vi "FPGA_PPG_query_command.vi"(0 "resource_in":refnum<visa-resource-name>, 2 "mem_addr":u32, 5 "error in (no error)":errorcluster) -> (14 "resource_out":refnum<visa-resource-name>, 16 "command":string, 19 "error out":errorcluster)   [LabVIEW 2014, in "NI-FPGA_PPG_Driver.lvlib"]
doc: "Queries the command specified by the address.\n\nContact: Falk Ziegler, eMail: ziegler@physik.uni-greifswald.de"
uses:
  NI-FPGA_PPG_Driver.lvlib
  <vilib>/rvi/interface/nirviReadWriteControl/nirviReadWriteControl.xnode
  <vilib>/rvi/interface/nirviMethod/nirviMethod.xnode
  FPGA_PPG_action_type.ctl
  FPGA_PPG_error_type.ctl
  FPGA_PPG_vi_ref.ctl
  D:/Workspace/PyCharm/Tilda/TildaTarget/Labview14/FPGA Bitfiles/TiTaProj_COF_PPG_100MHz.lvbitx
  <vilib>/rvi/errors/niLvFpgaMergeErrorWithErrorCode.vi
panel:
  in  "errorCodes":T1=enum."can't change state while pattern output is in progress"
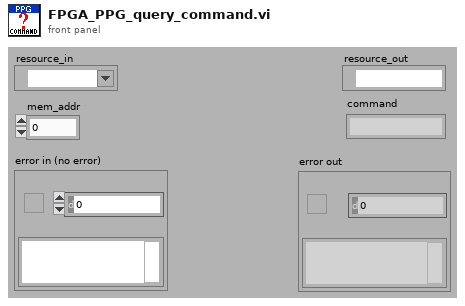
[diagram p1: front panel]
types:
  T1 = typedef "NI-FPGA_PPG_Driver.lvlib/FPGA_PPG_error_type.ctl" = enum16{"no error", "resource not initialized (no commands and invalid mem address)", "wrong memory address (address > Nof commands)", "invalid time value (probably too short)", "cannot start FPGA because one or more errors occured", "FIFO (internal) empty unexpectedly", "DMA FIFO (download from host) full unexpectedly", "checking number of commands: failed", "unknown error 8", "unknown error 9", "unknown error 10", "unknown error 11", "unknown error 12", "unknown error 13", "unknown error 14", "unknown error 15", "unknown error 16", "unknown error 17", "unknown error 18", "unknown error 19", "can't change state while pattern output is in progress"}
  T2 = typedef "NI-FPGA_PPG_Driver.lvlib/FPGA_PPG_action_type.ctl" = enum16{"GET", "SET", "REMOVE"}
  T3 = typedef "NI-FPGA_PPG_Driver.lvlib/FPGA_PPG_vi_ref.ctl" = refnum<k20>
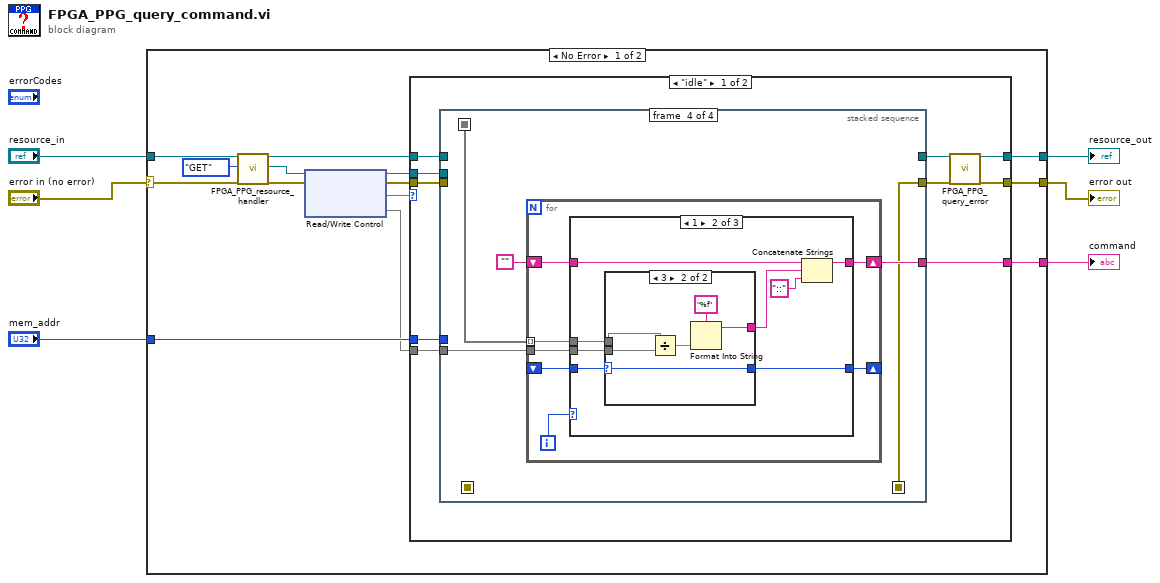
[diagram p0: block diagram]
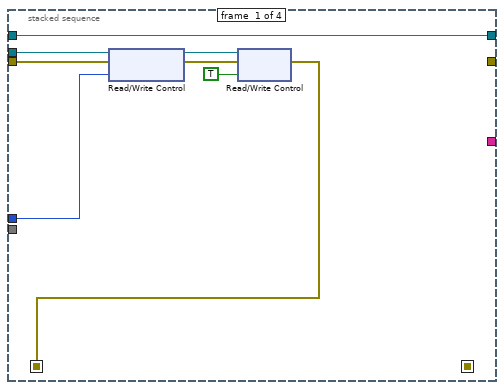
[diagram p2: hidden frame]
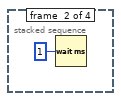
[diagram p3: hidden frame]
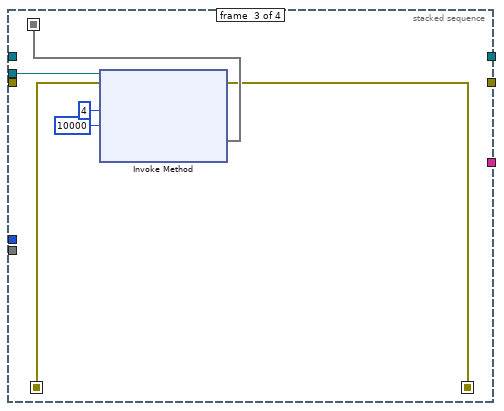
[diagram p4: hidden frame]
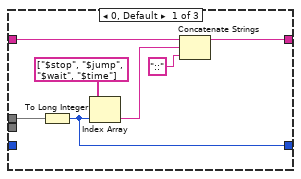
[diagram p5: hidden frame]
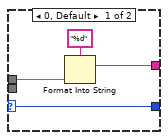
[diagram p6: hidden frame]
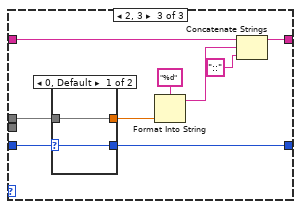
[diagram p7: hidden frame]
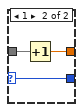
[diagram p8: hidden frame]
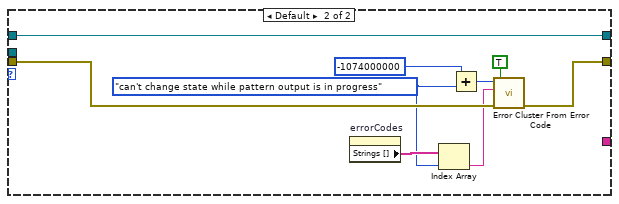
[diagram p9: hidden frame]
diagram:
  n1 = case shown="No Error" "error in (no error)" {
    selector: "error in (no error)" -> [w19 w107]
    tunnel: [w10 w107] -> w5
    tunnel: "resource_in" -> [w20 w106]
    tunnel: [w11 w106] -> w3
    tunnel: "mem_addr" -> [w13 _]
    tunnel: [w12 _] -> w1
    frame No Error {
      n2 = call "FPGA_PPG_resource_handler.vi"("resource_in"=w20, "action"=FPGA_PPG_action_type."GET", "error in (no error)"=w19) -> ("resource_out"=w16:refnum<visa-resource-name>, "FPGA VI Reference Out"=w8:T3, "error out"=w18:errorcluster)  [unwired: 14 in]
      n3 = xnode ("Read/Write Control")("FPGA VI Reference In"=w8, "error in"=w18) -> ("FPGA VI Reference Out"=w15:T3, "error out"=w14:errorcluster, "state"=w17, "ticks_per_us"=w7)
      n4 = case shown="\"idle\"" w17 {
        tunnel: w16 -> [w27 w105]
        tunnel: w15 -> [w30 _]
        tunnel: w14 -> [w29 w104]
        tunnel: [w24 w105] -> w11
        tunnel: w13 -> [w28 _]
        tunnel: [w26 _] -> w12
        tunnel: [w23 w102] -> w10
        tunnel: w7 -> [w21 _]
        frame "idle" {
          n5 = stacked-sequence {
            seq-local: [w31 _ _ _] -> [_ _ w44 _]
            seq-local: [_ _ w41 _] -> [_ _ _ w50]
            seq-local: [_ _ w40 _] -> [_ _ _ w47]
            tunnel: w30 -> [w38 _ w45 _]
            tunnel: w29 -> [w37 _ _ _]
            tunnel: w28 -> [w36 _ _ _]
            tunnel: w27 -> [w32 _ _ _]
            tunnel: [w32 _ _ _] -> w25
            tunnel: [_ _ _ w48] -> w26
            tunnel: [_ _ _ w47] -> w22
            tunnel: w21 -> [_ _ _ w46]
            frame #0 {
              n6 = xnode ("Read/Write Control")("FPGA VI Reference In"=w38, "error in"=w37, "mem_addr"=w36) -> ("FPGA VI Reference Out"=w35:T3, "error out"=w34:errorcluster)
              n7 = xnode ("Read/Write Control")("FPGA VI Reference In"=w35, "error in"=w34, "query"=TRUE) -> ("error out"=w31:errorcluster)  [unwired: 1 out]
            }
            frame #1 {
              n8 = Wait (ms)(milliseconds to wait=u32 1) -> ()  [unwired: 1 out]
            }
            frame #2 {
              n9 = xnode ("Invoke Method")("FPGA VI Reference In"=w45, "error in"=w44, "Number of Elements"=u32 4, "Timeout (ms)"=10000) -> ("error out"=w40:errorcluster, "Data"=w41:void[])  [unwired: 2 out]
            }
            frame #3 {
              n10 = for {
                tunnel: w50 -> [w56] mode=indexing
                shift-right: [w54] -> w48
                shift-left: "" ("Empty String Constant") -> [w55]
                shift-right: [w52] -> _
                shift-left: _ -> [w53]
                tunnel: w46 -> [w51]
                i -> [w57]
                n11 = case shown="1" w57 {
                  tunnel: w56 -> [w61 w68 w85]
                  tunnel: w55 -> [w63 w72 w89]
                  tunnel: [w62 w70 w87] -> w54
                  tunnel: [w58 w66 w83] -> w52
                  tunnel: w53 -> [_ w69 w86]
                  tunnel: w51 -> [_ w65 _]
                  frame 0, Default {
                    n12 = To Long Integer(number=w61) -> (32bit integer=w58:i32)
                    n13 = Index Array(array=string[] ["$stop", "$jump", "$wait", "$time"], index=w58) -> (element=w60:string)
                    n14 = Concatenate Strings(w63, w60, "::" ("string")) -> (w62:string)
                  }
                  frame 1 {
                    n15 = case shown="3" w69 {
                      selector: w69 -> [w73 w78]
                      tunnel: w68 -> [w75 w82]
                      tunnel: [w74 w79] -> w67
                      tunnel: [w73 w78] -> w66
                      tunnel: w65 -> [_ w77]
                      frame 0, Default {
                        n16 = Format Into String(format string="%d", w75) -> (resulting string=w74:string)  [unwired: 2 in, 1 out]
                      }
                      frame 3 {
                        n17 = Divide(x=w82, y=w77) -> (x/y=w80:dbl)
                        n18 = Format Into String(format string="%f", w80) -> (resulting string=w79:string)  [unwired: 2 in, 1 out]
                      }
                    }
                    n19 = Concatenate Strings(w72, w67, "::" ("string")) -> (w70:string)
                  }
                  frame 2, 3 {
                    n20 = case shown="0, Default" w86 {
                      selector: w86 -> [w92 w94]
                      tunnel: w85 -> [w93 w95]
                      tunnel: [w93 w96] -> w84
                      tunnel: [w92 w94] -> w83
                      frame 0, Default {
                      }
                      frame 1 {
                        n21 = Increment(x=w95) -> (x+1=w96:dbl)
                      }
                    }
                    n22 = Format Into String(format string="%d", w84) -> (resulting string=w90:string)  [unwired: 2 in, 1 out]
                    n23 = Concatenate Strings(w89, w90, "::" ("string")) -> (w87:string)
                  }
                }
              }
            }
          }
          n24 = call "FPGA_PPG_query_error.vi"("resource_in"=w25, "error in (no error)"=w22) -> ("resource_out"=w24:refnum<visa-resource-name>, "error out"=w23:errorcluster)  [unwired: 16 in]
        }
        frame Default {
          w97 = FPGA_PPG_error_type."can't change state while pattern output is in progress" ("error code (0)")
          n25 = property on="errorCodes" class="Enum (strict)"() -> ("Strings []"=w101:string[])  [unwired: 2 in, 2 out]
          n26 = Index Array(array=w101, index=w97) -> (element=w100:string)
          n27 = Add(x=-1074000000 ("error code (0)"), y=w97) -> (x+y=w98:i32)
          n28 = call <vilib>:"Error Cluster From Error Code.vi"("show call chain? (False)"=TRUE, "error in (no error)"=w104, "error message (\"\")"=w100, "error code (0)"=w98) -> ("error out"=w102:errorcluster)  [unwired: 5 in]
        }
      }
    }
    frame Error {
    }
  }
  "error out" <- w5
  "resource_out" <- w3
  "command" <- w1
